vi "WPX App Data Files and Folders.vi"(9 "AppDataFolder":path, 10 "ApplicationName":string) -> (0 "DataFolder":path, 2 "INI File Path":path, 3 "Exec Log Path":path, 11 "system directory":path)   [LabVIEW 2017]
uses:
  <vilib>/Utility/sysdir.llb/System Directory Type.ctl
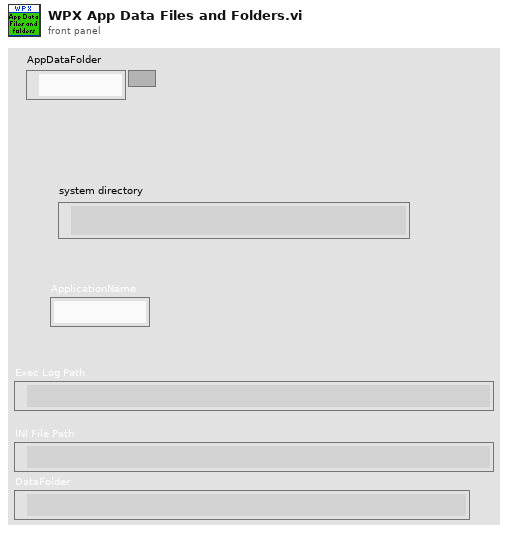
[diagram p1: front panel]
types:
  T1 = typedef "System Directory Type.ctl" = i32
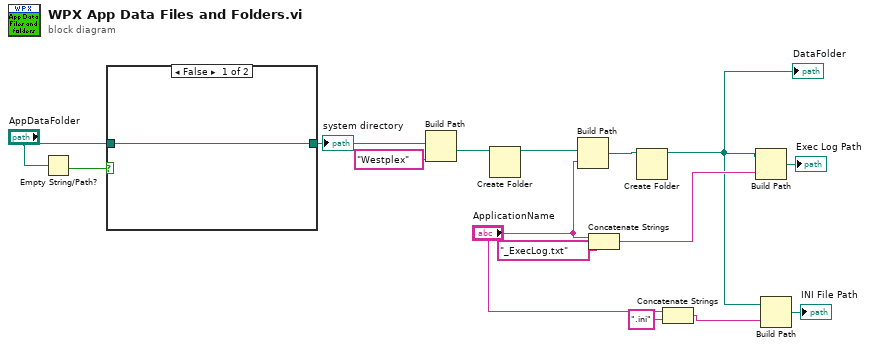
[diagram p0: block diagram]
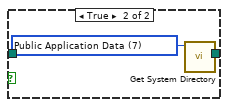
[diagram p2: hidden frame]
diagram:
  n1 = Empty String/Path?(string/path="AppDataFolder") -> (empty?=w2:bool)
  n2 = case shown="False" w2 {
    tunnel: [w16 w17] -> w15
    tunnel: "AppDataFolder" -> [w16 _]
    frame False {
    }
    frame True {
      w18 = T1 7 items=["User Home"=0, "User Desktop"=1, "User Documents"=2, "User Application Data"=3, "User Preferences"=4, "User Temporary"=5, "Public Documents"=6, "Public Application Data"=7, "Public Preferences"=8, "Public Cache"=13, "System Core Libraries"=9, "System Installed Libraries"=10, "Application Files"=11, "Boot Volume Root"=12] ("system directory type")
      n3 = call <vilib>:"Get System Directory.vi"("system directory type"=w18) -> ("system directory"=w17:path)  [unwired: 10 in]
    }
  }
  "system directory" <- w15
  n4 = Build Path(base path=w15, name or relative path="Westplex") -> (appended path=w6:path)
  n5 = Create Folder(path (use dialog)=w6) -> (created path=w5:path)  [unwired: 2 in, 2 out]
  n6 = Build Path(base path=w5, name or relative path="ApplicationName") -> (appended path=w4:path)
  n7 = Concatenate Strings("ApplicationName", "_ExecLog.txt" ("string")) -> (w12:string)
  n8 = Create Folder(path (use dialog)=w4) -> (created path=w3:path)  [unwired: 2 in, 2 out]
  "DataFolder" <- w3
  n9 = Concatenate Strings("ApplicationName", ".ini" ("string")) -> (w8:string)
  n10 = Build Path(base path=w3, name or relative path=w12) -> (appended path=→"Exec Log Path":path)
  n11 = Build Path(base path=w3, name or relative path=w8) -> (appended path=→"INI File Path":path)
